vi "Get Ctls Recursive.vi"(8 "Error In":errorcluster, 10 "Traverse Clusters (F)":bool=TRUE, 11 "Ctls":refnum<vi>[](array[refnum])) -> (0 "Error Out":errorcluster, 3 "Recursive All Ctls":refnum<vi>[](array[refnum]))   [LabVIEW 2015, in "UIM.lvclass"]
uses:
  UIM.lvclass
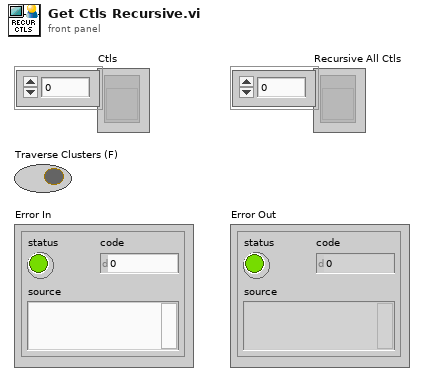
[diagram p1: front panel]
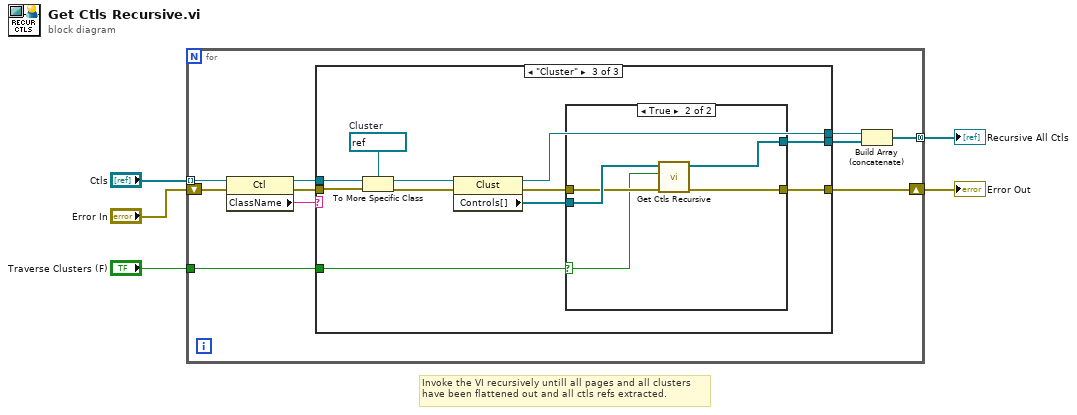
[diagram p0: block diagram]
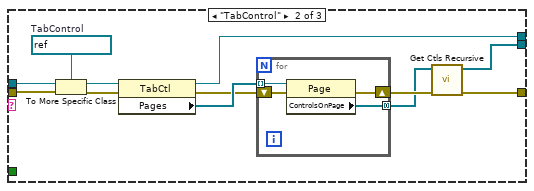
[diagram p3: hidden frame]
diagram:
  # "Invoke the VI recursively untill all pages and all clusters\nhave been flattened out and all ctls refs extracted."
  n1 = for {
    tunnel: "Ctls" -> [w15] mode=indexing
    tunnel: [w8] -> w4 mode=concatenating
    shift-right: [w7] -> w5
    shift-left: "Error In" -> [w12]
    tunnel: "Traverse Clusters (F)" -> [w6]
    n2 = property class="Ctl"(reference=w15, error in=w12) -> (reference out=w13:refnum<vi>, error out=w11:errorcluster, "ClassName"=w14:string)
    n3 = case shown="\"Cluster\"" w14 {
      tunnel: w13 -> [w17 w28 w43]
      tunnel: w11 -> [w16 w27 w42]
      tunnel: [w17 w22 w35] -> w10
      tunnel: [_ w19 w36] -> w9
      tunnel: [w16 w18 w37] -> w7
      tunnel: w6 -> [_ _ w34]
      frame Default {
        # "If not TAB or CLUSTER do nothing"
      }
      frame "TabControl" {
        w29 = refnum<vi> refnum  # TabControl
        n4 = To More Specific Class(target class=w29, reference=w28, error in=w27) -> (specific class reference=w26:refnum<vi>, error out=w25:errorcluster)
        n5 = property class="TabCtl"(reference=w26, error in=w25) -> (reference out=w22:refnum<vi>, error out=w23:errorcluster, "Pages"=w24:refnum<vi>[])
        n6 = for {
          tunnel: w24 -> [w33] mode=indexing
          shift-right: [w31] -> w21
          shift-left: w23 -> [w32]
          tunnel: [w30] -> w20 mode=concatenating
          n7 = property class="Page"(reference=w33, error in=w32) -> (error out=w31:errorcluster, "ControlsOnPage"=w30:refnum<vi>[])  [unwired: 1 out]
        }
        n8 = call "Get Ctls Recursive.vi"("Error In"=w21, "Ctls"=w20) -> ("Error Out"=w18:errorcluster, "Recursive All Ctls"=w19:refnum<vi>[])  [unwired: 8 in]
      }
      frame "Cluster" {
        w44 = refnum<vi> refnum  # Cluster
        n9 = To More Specific Class(target class=w44, reference=w43, error in=w42) -> (specific class reference=w41:refnum<vi>, error out=w40:errorcluster)
        n10 = property class="Clust"(reference=w41, error in=w40) -> (reference out=w35:refnum<vi>, error out=w38:errorcluster, "Controls[]"=w39:refnum<vi>[])
        n11 = case shown="True" w34 {
          selector: w34 -> [_ w46]
          tunnel: w39 -> [_ w50]
          tunnel: w38 -> [w45 w49]
          tunnel: [w45 w48] -> w37
          tunnel: [_ w47] -> w36
          frame False {
          }
          frame True {
            n12 = call "Get Ctls Recursive.vi"("Error In"=w49, "Traverse Clusters (F)"=w46, "Ctls"=w50) -> ("Error Out"=w48:errorcluster, "Recursive All Ctls"=w47:refnum<vi>[])  [unwired: 7 in]
          }
        }
      }
    }
    n13 = Build Array (concatenate)(w10, w9) -> (w8:refnum<vi>[])
  }
  "Error Out" <- w5
  "Recursive All Ctls" <- w4
